vi "Get Exponent of a Number (I32).vi"(9 "Input Valid":bool=TRUE, 10 "Binary Number":i32 format="%.0b") -> (1 "Output Valid":bool, 2 "Exponent":u8, 5 "Binary Number":i32 format="%032b")   [LabVIEW 2010]
uses:
  <vilib>/rvi/FXPMathLib/basic elements/FxpDiscreteDelay/XNode/nifxpmath_DiscreteDelay.xnode
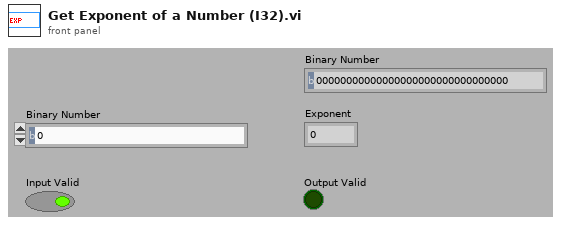
[diagram p1: front panel]
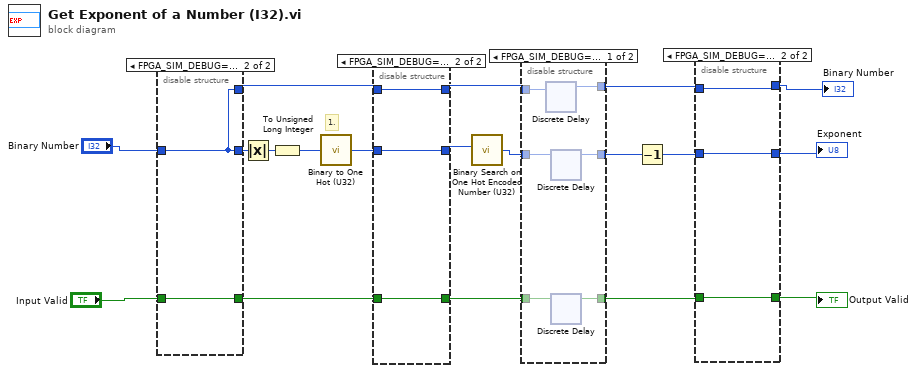
[diagram p0: block diagram]
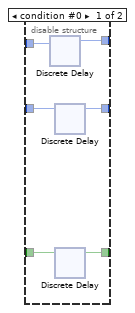
[diagram p2: hidden frame]
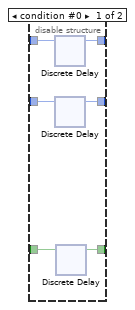
[diagram p4: hidden frame]
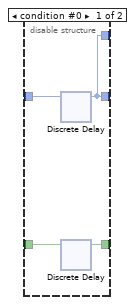
[diagram p5: hidden frame]
diagram:
  # "1."
  n1 = disable-structure shown="FPGA_SIM_DEBUG==TRUE" {
    disable-tunnel: [w20 w88] -> w19
    disable-tunnel: "Input Valid" -> [w23 w89]
    disable-tunnel: [w22 w89] -> w17
    disable-tunnel: "Binary Number" -> [w21 w88]
    disable-tunnel: [w20 w88] -> w12
    frame condition #0 {
      n2 = xnode "Discrete Delay"("D"=w21) -> ("Q"=w20:i32)
      n3 = xnode "Discrete Delay"("D"=w23) -> ("Q"=w22:bool)
    }
    frame condition #1 (active) {
    }
  }
  n4 = Absolute Value(x=w19) -> (abs(x)=w9:i32)
  n5 = To Unsigned Long Integer(number=w9) -> (unsigned 32bit integer=w8:u32)
  n6 = call "Binary to One Hot (U32).vi"("Binary Number"=w8) -> ("One Hot Encoded Number"=w15:u32)  [unwired: 14 in]
  n7 = disable-structure shown="FPGA_SIM_DEBUG==TRUE" {
    disable-tunnel: w17 -> [w95 w193]
    disable-tunnel: [w94 w193] -> w16
    disable-tunnel: w15 -> [w93 w194]
    disable-tunnel: [w92 w194] -> w14
    disable-tunnel: w12 -> [w91 w192]
    disable-tunnel: [w90 w192] -> w11
    frame condition #0 {
      n8 = xnode "Discrete Delay"("D"=w91) -> ("Q"=w90:i32)
      n9 = xnode "Discrete Delay"("D"=w93) -> ("Q"=w92:u32)
      n10 = xnode "Discrete Delay"("D"=w95) -> ("Q"=w94:bool)
    }
    frame condition #1 (active) {
    }
  }
  n11 = call "Binary Search on One Hot Encoded Number (U32).vi"("One Hot Encoded Number"=w14) -> ("Binary Number"=w13:u8)  [unwired: 14 in]
  n12 = disable-structure shown="FPGA_SIM_DEBUG==FALSE, default" {
    disable-tunnel: [w200 w299] -> w6
    disable-tunnel: [w199 w298] -> w4
    disable-tunnel: w16 -> [w198 w298]
    disable-tunnel: w13 -> [w197 w299]
    disable-tunnel: w11 -> [w196 w297]
    disable-tunnel: [w195 w297] -> w7
    frame condition #0 {
      n13 = xnode "Discrete Delay"("D"=w196) -> ("Q"=w195:i32)
      n14 = xnode "Discrete Delay"("D"=w197) -> ("Q"=w200:u8)
      n15 = xnode "Discrete Delay"("D"=w198) -> ("Q"=w199:bool)
    }
    frame condition #1 (active) {
    }
  }
  n16 = Decrement(x=w6) -> (x-1=w5:u8)
  n17 = disable-structure shown="FPGA_SIM_DEBUG==TRUE" {
    disable-tunnel: [w305 w404] -> w2
    disable-tunnel: [w304 w403] -> w3
    disable-tunnel: w4 -> [w303 w403]
    disable-tunnel: w5 -> [w302 w404]
    disable-tunnel: w7 -> [w301 w402]
    disable-tunnel: [w300 w402] -> w1
    frame condition #0 {
      n18 = xnode "Discrete Delay"("D"=w301) -> ("Q"=w300:i32)
      n19 = xnode "Discrete Delay"("D"=w302) -> ("Q"=w305:u8)
      n20 = xnode "Discrete Delay"("D"=w303) -> ("Q"=w304:bool)
    }
    frame condition #1 (active) {
    }
  }
  "Exponent" <- w2
  "Output Valid" <- w3
  "Binary Number" <- w1
